vi "Configure String Parameter.vi"(6 "value":string, 7 "process number":u8, 8 "error in (no error)":errorcluster, 9 "parameter number":u8, 10 "node":u8, 11 "ProPar in":refnum<class "PL Bronkhorst ProPar.lvclass">) -> (0 "error out":errorcluster, 3 "ProPar out":refnum<class "PL Bronkhorst ProPar.lvclass">)   [LabVIEW 2015, in "PL Bronkhorst ProPar.lvclass"]
doc: "Configures specified string <b>parameter</b> of the specified <b>node</b>."
uses:
  PL Bronkhorst ProPar.lvclass
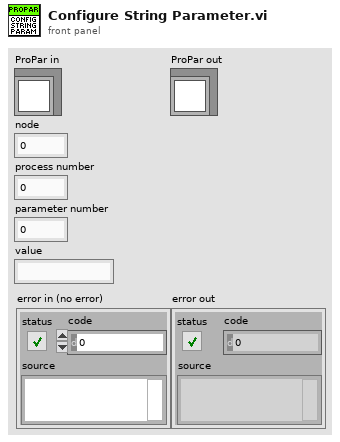
[diagram p1: front panel]
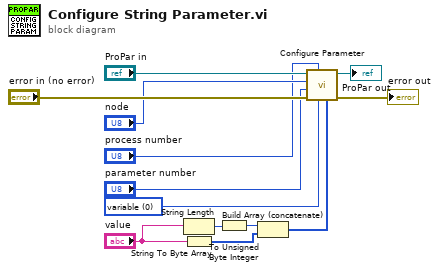
[diagram p0: block diagram]
diagram:
  w1 = u8 0 items=["variable"=0, "1"=1, "2"=2, "4"=4] ("value byte count")
  n1 = String Length(string="value") -> (length=w5:i32)
  n2 = String To Byte Array(string="value") -> (unsigned byte array=w3:u8[])
  n3 = To Unsigned Byte Integer(number=w5) -> (unsigned 8bit integer=w4:u8)
  n4 = Build Array (concatenate)(w4, w3) -> (w2:u8[])
  n5 = call "Configure Parameter.vi"("value"=w2, "value byte count"=w1, "process number"="process number", "error in (no error)"="error in (no error)", "parameter number"="parameter number", "node"="node", "ProPar in"="ProPar in") -> ("error out"=→"error out":errorcluster, "ProPar out"=→"ProPar out":refnum<class "PL Bronkhorst ProPar.lvclass">)  [unwired: 3 in]
